vi "Get SMARTDAC Type.vi"(8 "error in (no error)":errorcluster, 11 "VISA resource name":refnum<visa-resource-name>) -> (0 "error out":errorcluster, 2 "SMARTDAC+ Type":u16(ring) items=["Unknown", "GX10", "GX20", "GP10", "GP20", "GM10"], 3 "VISA resource name out":refnum<visa-resource-name>)   [LabVIEW 2020, in "Yokogawa GX Series.lvlib"]
doc: "This VI logouts from the instrument. Then it can not re-login."
uses:
  <instrlib>/Yokogawa GX Series/Yokogawa GX Series.lvlib
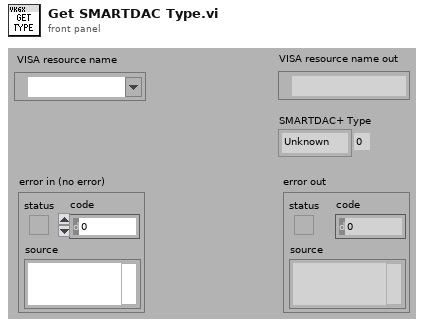
[diagram p1: front panel]
types:
  T1 = cluster{"User Name":string, "User ID":string, "Password":string, "Serial Auth Type (0: Not Auth)":u16, "SMARTDAC+ Type (0: Unknown)":u16, "Bluetooth Password":string}
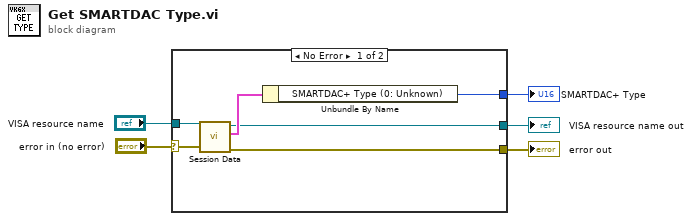
[diagram p0: block diagram]
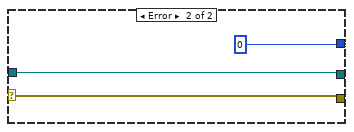
[diagram p2: hidden frame]
diagram:
  n1 = case shown="No Error" "error in (no error)" {
    selector: "error in (no error)" -> [w10 w14]
    tunnel: "VISA resource name" -> [w11 w13]
    tunnel: [w8 w14] -> w4
    tunnel: [w7 w13] -> w2
    tunnel: [w6 u16 0] -> w1
    frame No Error {
      n2 = call <instrlib>:"Session Data.vi"("error in (no error)"=w10, "VISA resource name"=w11) -> ("error out"=w8:errorcluster, "User Data Out"=w9:T1, "VISA resource name out"=w7:refnum<visa-resource-name>)  [unwired: 7 in]
      n3 = Unbundle By Name(w9) -> ("SMARTDAC+ Type (0: Unknown)"=w6:u16)
    }
    frame Error {
    }
  }
  "error out" <- w4
  "VISA resource name out" <- w2
  "SMARTDAC+ Type" <- w1
